vi "Step Flow.vi"(8 "error in (no error)":errorcluster, 11 "Numeric Limit Compare in":refnum<class "Numeric Limit Compare.lvclass">) -> (0 "error out":errorcluster, 3 "Numeric Limit Compare out":refnum<class "Numeric Limit Compare.lvclass">)   [LabVIEW 2015, in "Numeric Limit Compare.lvclass"]
uses:
  Numeric Limit Compare.lvclass
  classes/Step/Execution/StepState.ctl
  classes/Step/Execution/Step Status.ctl
  classes/Step/Execution/Step Flow Control.ctl
  Numeric Limit Compare.lvclass/Numeric Limit Compare.ctl
  classes/Step/Execution/Step.lvclass
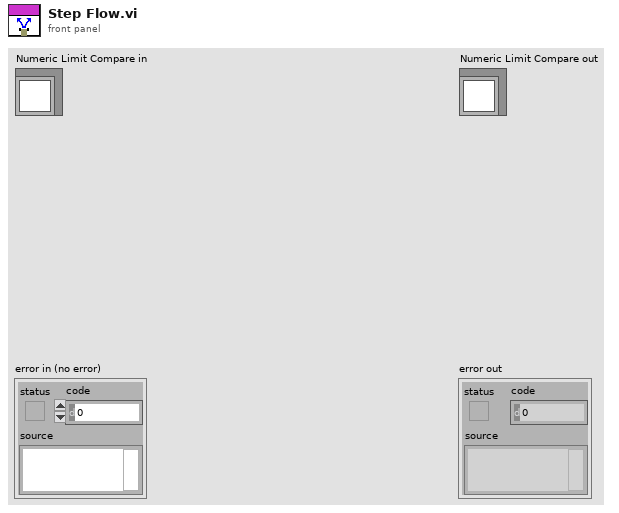
[diagram p1: front panel]
types:
  T1 = typedef "Step.lvclass/Step Status.ctl" = enum16{"Start", "Passed", "Failed", "Error", "Done", "Terminated", "Skipped", "Running"}
  T2 = typedef "Step.lvclass/StepState.ctl" = cluster{"Step State":T1, "Flow Control":T3, "Jump Index":i32, "Done":bool}
  T3 = typedef "Step.lvclass/Step Flow Control.ctl" = enum16{"Next Step", "Jump"}
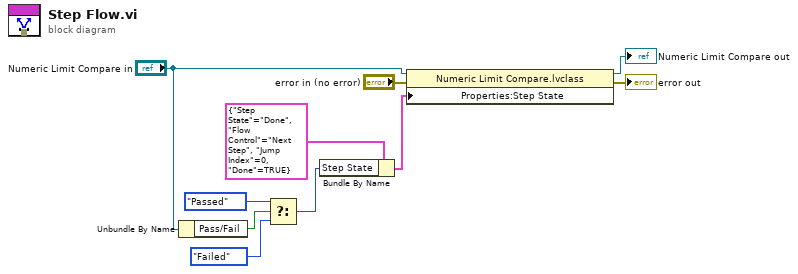
[diagram p0: block diagram]
diagram:
  n1 = Unbundle By Name("Numeric Limit Compare in") -> ("Pass/Fail"=w2:bool)
  n2 = Select(t=Step_Status."Passed" ("Step State"), s=w2, f=Step_Status."Failed" ("Step State")) -> (s? t:f=w4:T1)
  n3 = Bundle By Name(cluster=T2 {"Step State"=enum."Done", "Flow Control"=enum."Next Step", "Jump Index"=0, "Done"=TRUE} ("Step State"), "Step State"=w4) -> (w5:T2)
  n4 = property class="Numeric Limit Compare.lvclass"(reference="Numeric Limit Compare in", error in="error in (no error)", "Properties:Step State"=w5) -> (reference out=→"Numeric Limit Compare out":refnum<class "Numeric Limit Compare.lvclass">, error out=→"error out":errorcluster)
